vi "Command (read & write) - SI.vi"(7 "timeout ms (100)":i32=100, 8 "error in (no error)":errorcluster, 9 "Input Usage State":i32, 10 "IP":string, 11 "connection ID in":refnum<k16>) -> (0 "error out":errorcluster, 2 "Input Usage State":i32, 3 "connection ID out":refnum<k16>)   [LabVIEW 2016, in "SMD-7615.lvlib" / "eSCL.lvlib"]
doc: "SI - Enable Input Usage\nSets or requests the usage of the Enable input. Input X3 is the default Enable input on all drives, however IN3 on SE, QE and Si drives may also be designated as the Enable input (see below). If an external Enable function is not needed input X3 and/or IN3 can be defined solely as a general purpose input. In this scenario only the ME and MD commands will enable and disable the drive, respectively. When using the brake output (see BO, BD and BE commands) the disabling of the drive is delayed by the time value set using the BD command.\n\nSI1: Drive is enabled when X3 is open (inactive, high).\nSI2: Drive is enabled when X3 is closed (active, low).\nSI3: Neither X3 nor IN3 is used for enabling/disabling the drive, but as general purpose inputs.\nSI4: Drive is enabled when IN3 is open (inactive, high). (SE, QE, and Si drives only).\nSI5: Drive is enabled when IN3 is closed (active, low). (SE, QE, and Si drives only)."
uses:
  eSCL.lvlib
  I32 Command and Param.ctl
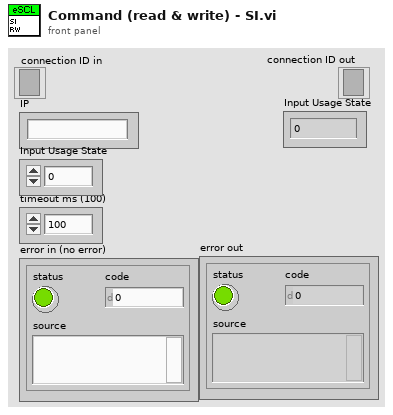
[diagram p1: front panel]
types:
  T1 = typedef "SMD-7615.lvlib/eSCL.lvlib/I32 Command and Param.ctl" = cluster{"Command":string, "I32 Parameler":i32, "I32 Parameler Default":i32, "I32 Parameler Coerece Upper":i32, "I32 Parameler Coerece Lower":i32}
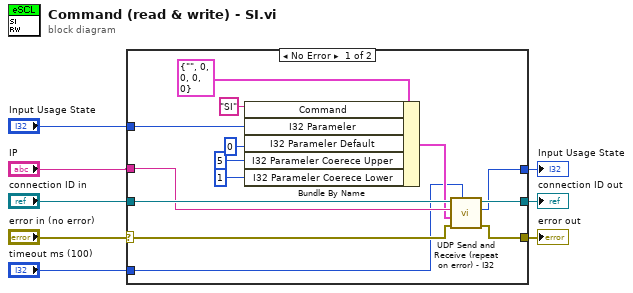
[diagram p0: block diagram]
diagram:
  n1 = case shown="No Error" "error in (no error)" {
    selector: "error in (no error)" -> [w16 w23]
    tunnel: "connection ID in" -> [w19 w24]
    tunnel: [w14 w24] -> w3
    tunnel: [w13 w23] -> w2
    tunnel: "IP" -> [w18 _]
    tunnel: "timeout ms (100)" -> [w15 _]
    tunnel: [w12 _] -> w1
    tunnel: "Input Usage State" -> [w9 _]
    frame No Error {
      n2 = Bundle By Name(cluster=T1 {"Command"="", "I32 Parameler"=0, "I32 Parameler Default"=0, "I32 Parameler Coerece Upper"=0, "I32 Parameler Coerece Lower"=0} ("I32 Command & Param"), "Command"="SI", "I32 Parameler"=w9, "I32 Parameler Default"=0 ("DBL Parameler Default"), "I32 Parameler Coerece Upper"=5 ("DBL Parameler Coerece Upper"), "I32 Parameler Coerece Lower"=1 ("DBL Parameler Coerece Lower")) -> (w17:T1)
      n3 = call "UDP Send and Receive (repeat on error) - I32.vi"("timeout ms (100)"=w15, "error in (no error)"=w16, "I32 Command & Param"=w17, "IP"=w18, "connection ID in"=w19) -> ("error out"=w13:errorcluster, "I32 Param out"=w12:i32, "connection ID out"=w14:refnum<k16>)  [unwired: 4 in]
    }
    frame Error {
    }
  }
  "connection ID out" <- w3
  "error out" <- w2
  "Input Usage State" <- w1
